vi "Module Get Instance.vi"(8 "error in (no error)":errorcluster, 11 "Self in":variant) -> (0 "error out":errorcluster, 2 "Instance":T1, 3 "Self out":variant)   [LabVIEW 2022 SP3, in "Core.lvlib"]
uses:
  Core.lvlib
  Controls/Module Instance.ctl
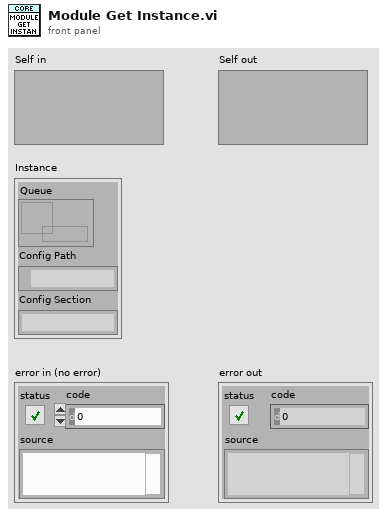
[diagram p1: front panel]
types:
  T1 = typedef "Core.lvlib/Module Instance.ctl" = cluster{"Queue":refnum<queue>, "Config Path":path, "Config Section":string}
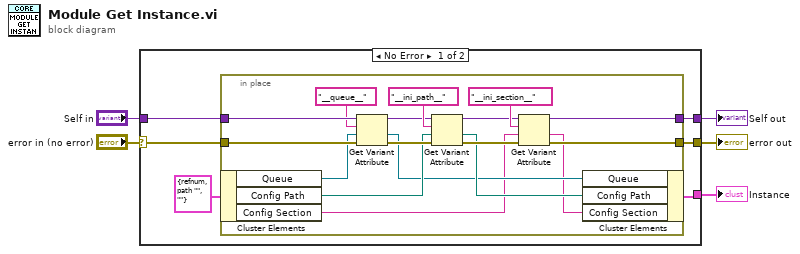
[diagram p0: block diagram]
diagram:
  n1 = case shown="No Error" "error in (no error)" {
    selector: "error in (no error)" -> [w11 w30]
    tunnel: "Self in" -> [w10 w29]
    tunnel: [w9 w30] -> w3
    tunnel: [w8 w29] -> w2
    tunnel: [w6 _] -> w1
    frame No Error {
      n2 = in-place {
        in-place-border: w11 -> [w28]
        in-place-border: w10 -> [w27]
        in-place-border: [w19] -> w9
        in-place-border: [w18] -> w8
        n3 = in-place-cluster #1(T1 {"Queue"=refnum, "Config Path"=path "", "Config Section"=""} ("Module Data")) -> ("Queue"=w17:refnum<queue>, "Config Path"=w16:path, "Config Section"=w13:string)
        n4 = Get Variant Attribute(Variant=w27, name="__queue__", default value (empty Variant)=w17, error in=w28) -> (duplicate Variant=w24:variant, value=w14:refnum<queue>, error out=w23:errorcluster)  [unwired: 1 out]
        n5 = Get Variant Attribute(Variant=w24, name="__ini_path__", default value (empty Variant)=w16, error in=w23) -> (duplicate Variant=w21:variant, value=w15:path, error out=w20:errorcluster)  [unwired: 1 out]
        n6 = Get Variant Attribute(Variant=w21, name="__ini_section__", default value (empty Variant)=w13, error in=w20) -> (duplicate Variant=w18:variant, value=w12:string, error out=w19:errorcluster)  [unwired: 1 out]
        n7 = in-place-cluster #1("Queue"=w14, "Config Path"=w15, "Config Section"=w12) -> (w6:T1)
      }
    }
    frame Error {
    }
  }
  "Self out" <- w2
  "error out" <- w3
  "Instance" <- w1
